vi "abcLookUp.vi"(9 "decoded message in":string, 10 "abc array of clusters":cluster{string, string}[](array[cluster]), 11 "Result String":string) -> (1 "String 2":string, 2 "decoded message out":string, 3 "String":string)   [LabVIEW 2017]
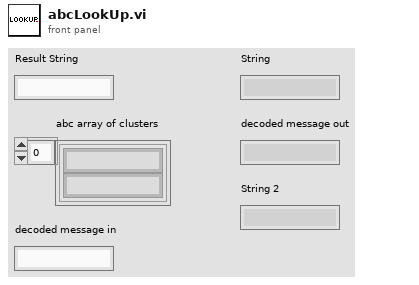
[diagram p1: front panel]
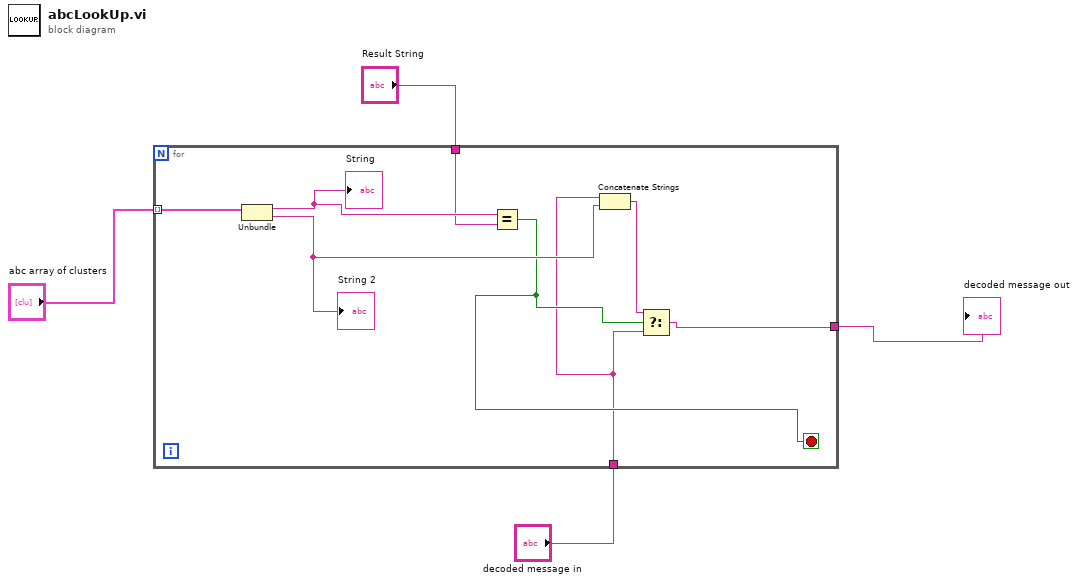
[diagram p0: block diagram]
diagram:
  n1 = for {
    tunnel: "abc array of clusters" -> [w12] mode=indexing
    tunnel: [w7] -> w2
    tunnel: "decoded message in" -> [w5]
    tunnel: "Result String" -> [w6]
    stop <- w8 stop-if-true
    n2 = Unbundle(w12) -> (w11:string, w10:string)
    "String" <- w11
    "String 2" <- w10
    n3 = Equal?(x=w11, y=w6) -> (x = y?=w8:bool)
    n4 = Concatenate Strings(w5, w10) -> (w9:string)
    n5 = Select(t=w9, s=w8, f=w5) -> (s? t:f=w7:string)
  }
  "decoded message out" <- w2
